vi "Homing.vi"(7 "Offset Home 2 RCM":dbl[](array[numeric])=[0.0, 0.0, 0.0, 0.0], 8 "error in":errorcluster, 9 "Stage PID Cluster":T2={"Stage Z PID"={"Kp"=0.0005, "Kd"=0.001, "Ki"=0.0}, "Stage Y PID"={"Kp"=0.0003, "Kd"=0.01, "Ki"=0.0}, "Stage X PID"={"Kp"=0.0003, "Kd"=0.01, "Ki"=0.0}}, 10 "L1 to L4 PID Cluster":T1={"L1 PID Gains"={"Kp"=0.005, "Kd"=0.5, "Ki"=0.0005}, "L2 PID Gains"={"Kp"=0.01, "Kd"=1.0, "Ki"=0.005}, "L3 PID Gains"={"Kp"=0.05, "Kd"=1.0, "Ki"=0.0005}, "L4 PID Gains"={"Kp"=0.1, "Kd"=0.1, "Ki"=0.0005}}, 11 "FPGA VI Reference In":refnum<k20>) -> (0 "error out":errorcluster, 1 "Last Stage Posit":dbl[](array[numeric]), 2 "Last L1 to L4 Posit":dbl[](array[numeric]), 3 "FPGA VI Reference Out":refnum<k20>)   [LabVIEW 2016]
uses:
  <vilib>/Platform/TimedLoop/XDataNode/timing_clust.ctl
  <vilib>/Platform/TimedLoop/XDataNode/nitl_modes.ctl
  <vilib>/Platform/TimedLoop/XDataNode/wakeup.ctl
  Library/KevinLibraryAll/labview2010/kevLib2010/Simple Filters/kDelay.vi
  Global Variables.vi
  <vilib>/Utility/error.llb/Error Cluster From Error Code.vi
  <vilib>/rvi/errors/niLvFpgaAdjustHostInterfaceError.vi
  <vilib>/platform/TimedLoop/XDataNode/XDataNode.xnode
  <vilib>/rvi/interface/nirviReadWriteControl/nirviReadWriteControl.xnode
  FPGA Bitfiles/IRISSTrack_FPGATarget2_IRISSFPGAIORIO_4NTO9ubhv-c.lvbitx
  IRISS_FPGA_IO_RIO.vi
  <vilib>/Platform/TimedLoop/XDataNode/XDNodeRunTimeDep.lvlib
  Library/KevinLibraryAll/labview2010/kevLib2010.lvlib
  Library/KevinLibraryAll/labview2011/kevLib2011.lvlib
  Library/KevinLibraryAll/labview/KevLib01.lvlib
  Library/jmslib.lvlib
  NiFpgaLv.dll
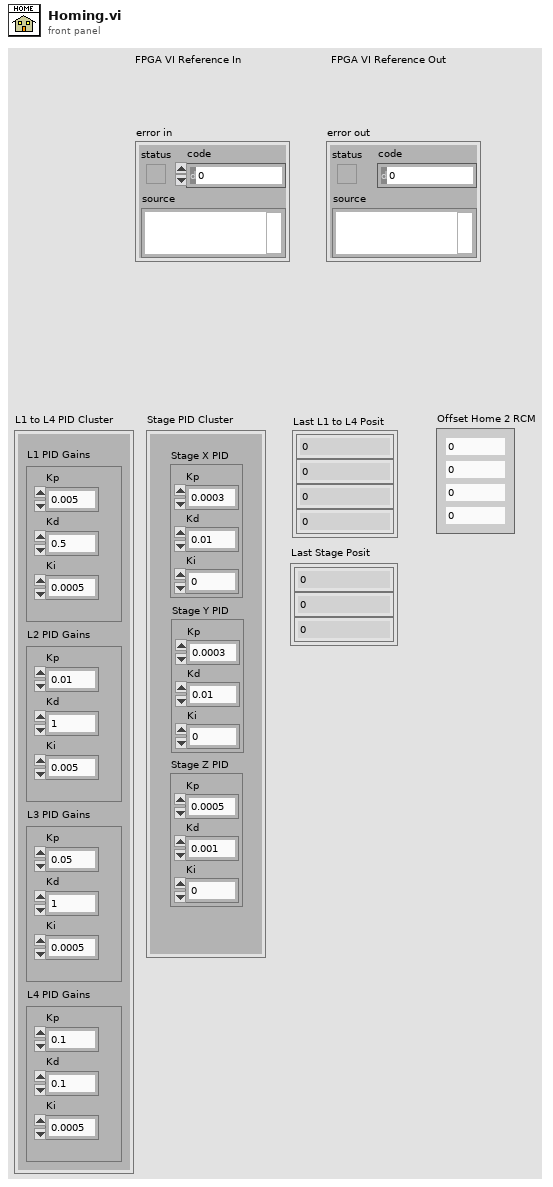
[diagram p1: front panel]
types:
  T1 = cluster{"L1 PID Gains":cluster{"Kp":dbl, "Kd":dbl, "Ki":dbl}, "L2 PID Gains":cluster{"Kp":dbl, "Kd":dbl, "Ki":dbl}, "L3 PID Gains":cluster{"Kp":dbl, "Kd":dbl, "Ki":dbl}, "L4 PID Gains":cluster{"Kp":dbl, "Kd":dbl, "Ki":dbl}}
  T2 = cluster{"Stage Z PID":cluster{"Kp":dbl, "Kd":dbl, "Ki":dbl}, "Stage Y PID":cluster{"Kp":dbl, "Kd":dbl, "Ki":dbl}, "Stage X PID":cluster{"Kp":dbl, "Kd":dbl, "Ki":dbl}}
  T3 = typedef "XDNodeRunTimeDep.lvlib/timing_clust.ctl" = cluster{"Expected End [f-1]":u64, "Actual End [f-1]":u64, "Finished Late? [f-1]":bool, "Expected End [i-1]":u64, "Actual End [i-1]":u64, "Finished Late? [i-1]":bool, "Expected Start [i]":u64, "Actual Start [i]":u64, "Expected Start [f]":u64, "Actual Start [f]":u64, "Source Name":string, "Structure Name":string, "Period":i64, "Deadline":i64, "Offset":i64, "Start":i64, "Priority":i32, "Timeout":i32, "Mode":T4, "Wakeup Reason":T5, "Error":errorcluster, "Source Type":string, "Secondary Source Type":string, "Global End Time":u64, "Global Start Time":u64, "Frame Duration":u64, "Iteration Duration":u64, "Assigned CPU":i32, "I/O Scan Engine Mode":u32}
  T4 = typedef "XDNodeRunTimeDep.lvlib/nitl_modes.ctl" = enum32{"No Change", "Process missed periods, maintain original phase", "Discard missed periods, maintain original phase", "Process missed periods, ignore original phase", "Discard missed periods, ignore original phase"}
  T5 = typedef "XDNodeRunTimeDep.lvlib/wakeup.ctl" = enum32{"Normal", "Aborted", "Asynchronous wakeup", "Timing source error", "Timed loop error", "Timeout"}
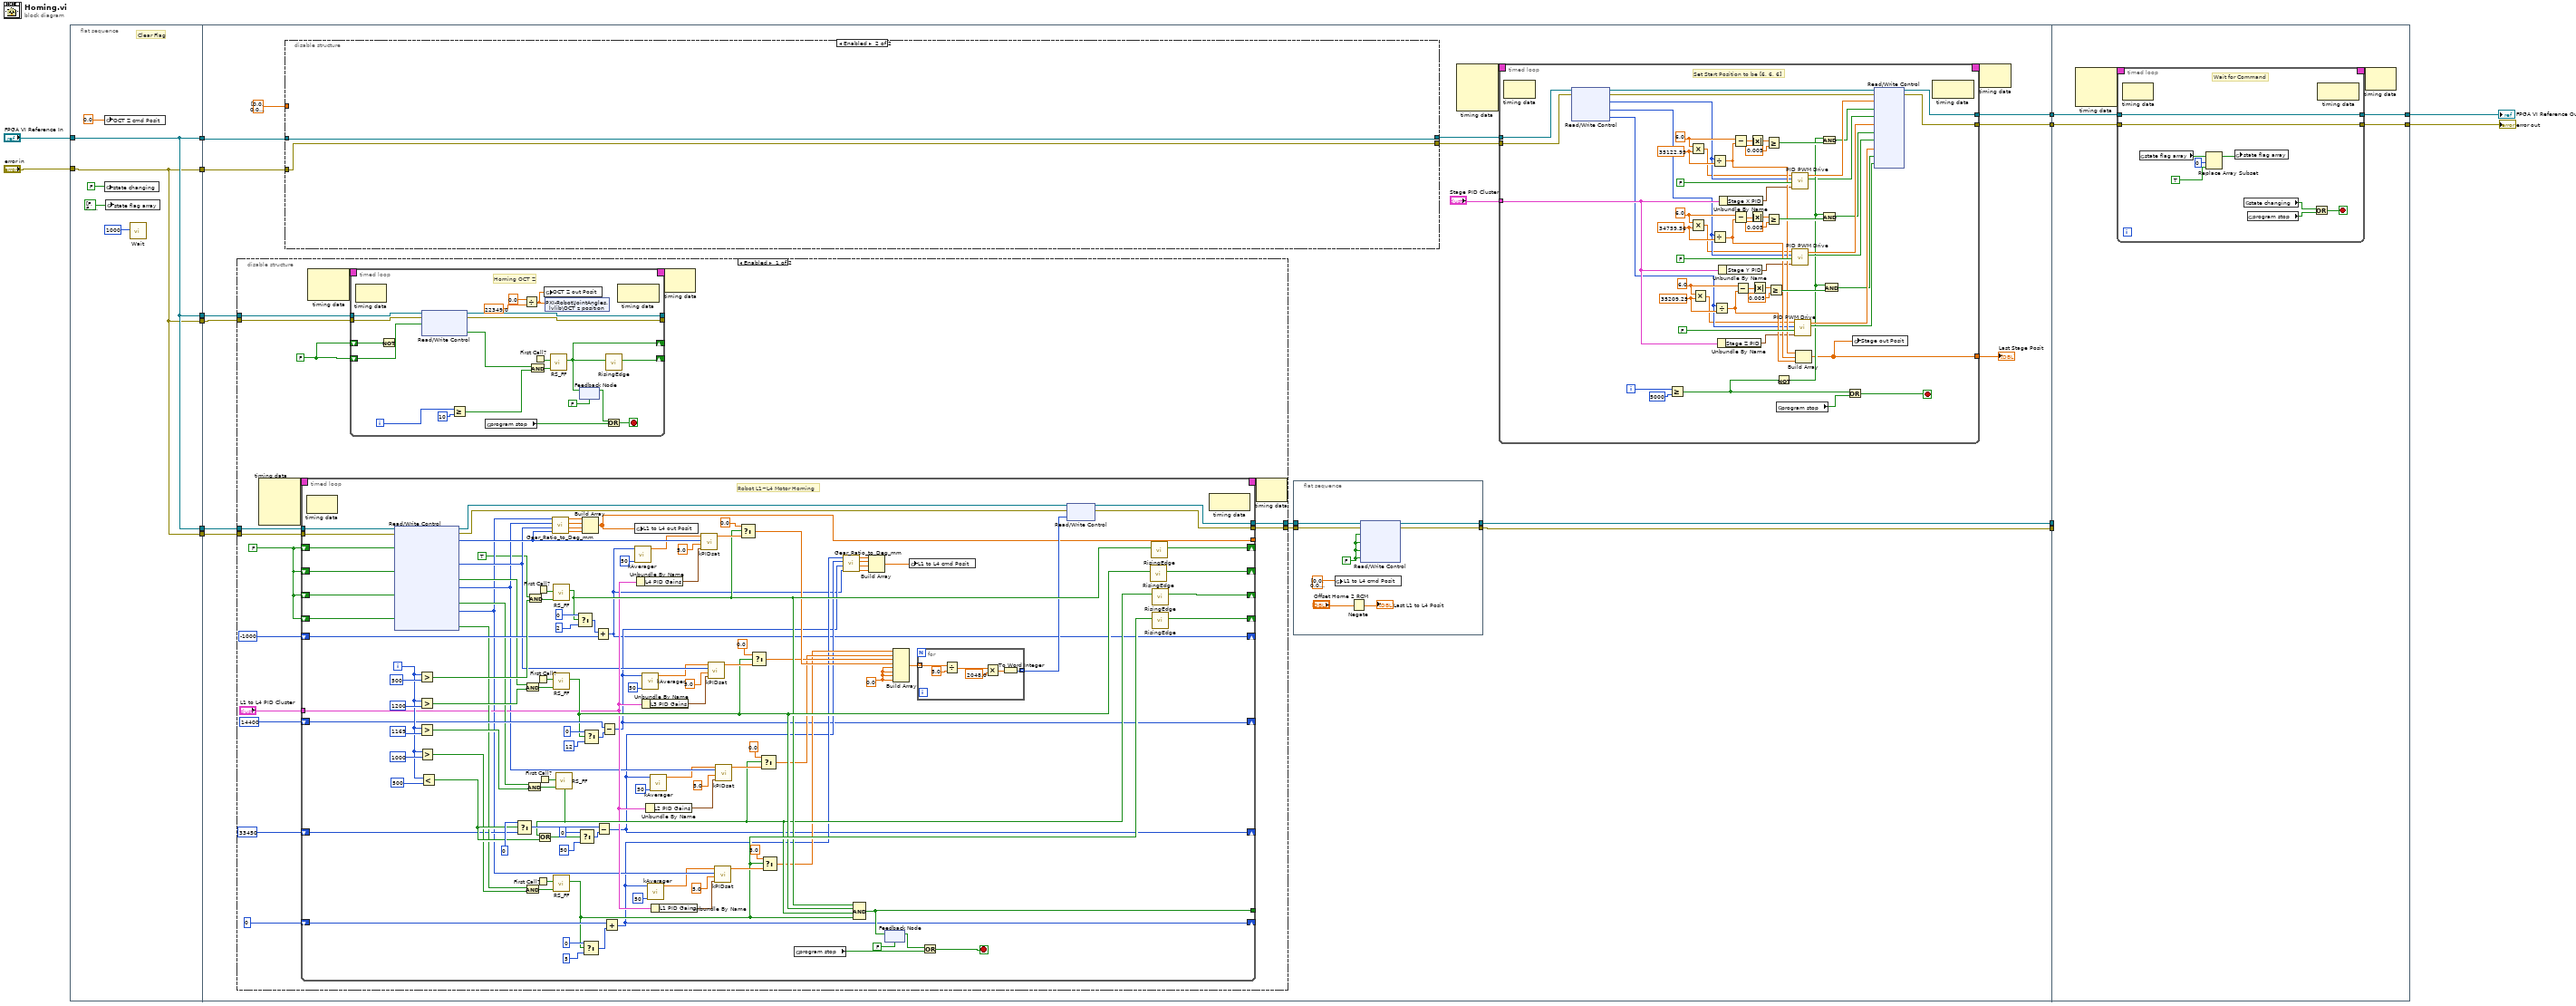
[diagram p0: block diagram]
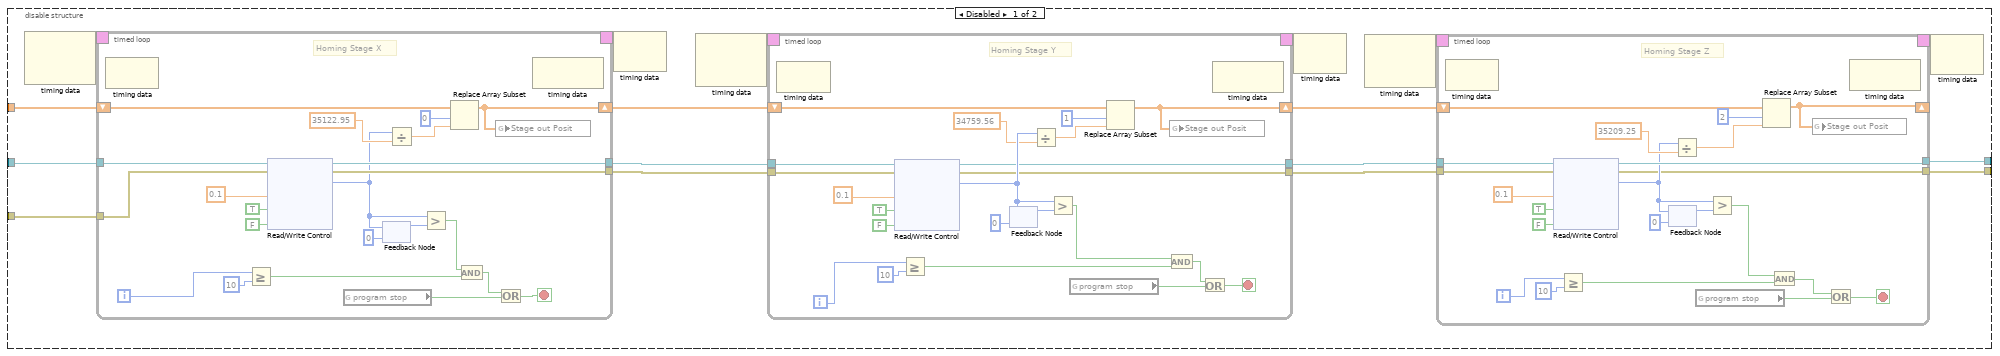
[diagram p3: hidden frame]
diagram:
  n1 = flat-sequence {
    tunnel: "FPGA VI Reference In" -> [w17]
    tunnel: "error in" -> [w16]
    tunnel: [w17] -> w14
    tunnel: [w17] -> w13
    tunnel: [w16] -> w12
    tunnel: [w16] -> w11
    tunnel: [w17] -> w6
    tunnel: [w16] -> w5
    tunnel: w14 -> [w37]
    tunnel: w13 -> [w36]
    tunnel: w12 -> [w35]
    tunnel: w11 -> [w34]
    tunnel: w6 -> [w33]
    tunnel: w5 -> [w32]
    tunnel: [w31] -> w4
    tunnel: [w30] -> w3
    tunnel: [w24] -> w2
    tunnel: [w23] -> w1
    tunnel: [w375] -> w8
    tunnel: [w374] -> w7
    tunnel: w4 -> [_]
    tunnel: w3 -> [_]
    tunnel: w2 -> [w373]
    tunnel: w1 -> [w372]
    frame #0 {
      # "Clear Flag"
      n2 = global write "Global Variables.vi" "OCT Z cmd Posit"(0.0) -> ()
      n3 = global write "Global Variables.vi" "state changing"(FALSE ("state changing")) -> ()
      n4 = global write "Global Variables.vi" "state flag array"(bool[] [FALSE, FALSE, FALSE, FALSE, FALSE, FALSE, FALSE, FALSE, FALSE] ("state flag array")) -> ()
      n5 = call "Wait"("Count(mSec)"=u32 1000 ("milliseconds to wait")) -> ()  [unwired: 1 out]
    }
    frame #1 {
      n6 = disable-structure shown="Enabled" {
        disable-tunnel: w36 -> [w52 _]
        disable-tunnel: w34 -> [w51 _]
        disable-tunnel: w33 -> [w50 _]
        disable-tunnel: w32 -> [w49 _]
        disable-tunnel: [w47 _] -> w22
        disable-tunnel: [w46 _] -> w21
        frame Enabled {
          w45 = FALSE ("Rising Edge")
          w48 = FALSE ("Rising Edge")
          n7 = node-c288() -> (w54:T3)  [unwired: 4 in]
          n8 = timed-loop {
            timing: w54 -> [_]
            timing-out: [_] -> w53
            tunnel: w52 -> [w171]
            tunnel: w51 -> [w170]
            shift-right: [w105] -> _
            shift-left: w45 -> [w169]
            shift-right: [w104] -> _
            shift-left: w45 -> [w168]
            shift-right: [w103] -> _
            shift-left: w45 -> [w167]
            shift-right: [w102] -> _
            shift-left: w45 -> [w166]
            shift-right: [w60] -> _
            shift-left: -1000 -> [w149]
            shift-right: [w61] -> _
            shift-left: 14400 -> [w141]
            shift-right: [w62] -> _
            shift-left: 33450 -> [w112]
            shift-right: [w63] -> _
            shift-left: 0 -> [w111]
            tunnel: [w106] -> _
            tunnel: [w86] -> w47
            tunnel: [w85] -> w46
            tunnel: "L1 to L4 PID Cluster" -> [w81]
            tunnel: [w59] -> _
            i -> [w151]
            stop <- w107 stop-if-true
            w97 = 0.0 ("element")
            # "Robot L1~L4 Motor Homing"
            n9 = node-c288() -> ()  [unwired: 1 in, 1 out]
            n10 = xnode "Read/Write Control"("FPGA VI Reference In"=w171, "error in"=w170, "Reset C1-4"=w169, "Reset C1-1"=w168, "Reset 3"=w167, "Reset 1"=w166) -> ("FPGA VI Reference Out"=w94:refnum<k20>, "error out"=w93:errorcluster, "32 bit Position C1-4"=w79:i32, "32 bit Position C1-1"=w78:i32, "Home L3"=w132:bool, "32 bit Position 3"=w77:i32, "Home L2"=w130:bool, "32 bit Position 1"=w76:i32, "Home L1"=w117:bool)  [unwired: 1 out]
            n11 = Greater?(x=w151, y=500) -> (0:w150:bool)
            n12 = Greater?(x=w151, y=1200) -> (0:w133:bool)
            n13 = Greater?(x=w151, y=1169) -> (0:w131:bool)
            n14 = Greater?(x=w151, y=1000) -> (0:w116:bool)
            n15 = Less?(x=w151, y=500) -> (x < y?=w123:bool)
            n16 = Select(t=0, s=w123, f=w112) -> (s? t:f=w128:i32)
            n17 = And(x=w132, y=w133) -> (x .and. y?=w142:bool)
            n18 = And(x=w117, y=w116) -> (x .and. y?=w118:bool)
            n19 = And(x=w130, y=w131) -> (x .and. y?=w135:bool)
            n20 = And(x=TRUE, y=w150) -> (x .and. y?=w162:bool)
            n21 = First Call?() -> (First Call?: T/F=w143:bool)
            n22 = First Call?() -> (First Call?: T/F=w119:bool)
            n23 = First Call?() -> (First Call?: T/F=w161:bool)
            n24 = First Call?() -> (First Call?: T/F=w134:bool)
            n25 = call "Gear_Ratio_to_Deg_mm.vi"("j4"=w79, "j3"=w78, "j2"=w77, "j1"=w76) -> ("theta 4"=w72:dbl, "theta 3"=w73:dbl, "theta 2"=w74:dbl, "theta 1"=w75:dbl)
            n26 = call "RS_FF.vi"("Set"=w162, "Reset"=w161) -> ("Result"=w99:bool)  [unwired: 9 in]
            n27 = call "RS_FF.vi"("Set"=w142, "Reset"=w143) -> ("Result"=w100:bool)  [unwired: 9 in]
            n28 = call "RS_FF.vi"("Set"=w118, "Reset"=w119) -> ("Result"=w101:bool)  [unwired: 9 in]
            n29 = call "RS_FF.vi"("Set"=w135, "Reset"=w134) -> ("Result"=w98:bool)  [unwired: 9 in]
            n30 = Or(x=w98, y=w123) -> (x .or. y?=w127:bool)
            n31 = Select(t=0, s=w99, f=2) -> (s? t:f=w163:i32)
            n32 = Select(t=0, s=w127, f=50) -> (s? t:f=w124:i32)
            n33 = Build Array(w75, w74, w73, w72) -> (w59:dbl[])
            n34 = Select(t=0, s=w101, f=5) -> (s? t:f=w122:i32)
            n35 = Select(t=0, s=w100, f=12) -> (s? t:f=w144:i32)
            n36 = Add(x=w163, y=w149) -> (x+y=w60:i32)
            n37 = Subtract(x=w128, y=w124) -> (x-y=w62:i32)
            n38 = Subtract(x=w141, y=w144) -> (x-y=w61:i32)
            n39 = Add(x=w111, y=w122) -> (x+y=w63:i32)
            n40 = call "kAverager.vi"("num avg"=50, "input"=w60) -> ("output"=w64:dbl)  [unwired: 9 in]
            n41 = global write "Global Variables.vi" "L1 to L4 out Posit"(w59) -> ()
            n42 = Unbundle By Name(w81) -> ("L4 PID Gains"=w84:cluster{"Kp":dbl, "Kd":dbl, "Ki":dbl})
            n43 = Unbundle By Name(w81) -> ("L3 PID Gains"=w83:cluster{"Kp":dbl, "Kd":dbl, "Ki":dbl})
            n44 = call "kAverager.vi"("num avg"=50, "input"=w61) -> ("output"=w65:dbl)  [unwired: 9 in]
            n45 = Unbundle By Name(w81) -> ("L2 PID Gains"=w82:cluster{"Kp":dbl, "Kd":dbl, "Ki":dbl})
            n46 = call "kAverager.vi"("num avg"=50, "input"=w63) -> ("output"=w67:dbl)  [unwired: 9 in]
            n47 = call "kAverager.vi"("num avg"=50, "input"=w62) -> ("output"=w66:dbl)  [unwired: 9 in]
            n48 = Unbundle By Name(w81) -> ("L1 PID Gains"=w80:cluster{"Kp":dbl, "Kd":dbl, "Ki":dbl})
            n49 = call "kPIDsat.vi"("PID Gains"=w84, "Sat Limit"=5.0, "Position"=w79, "Reference"=w64) -> ("Control"=w158:dbl)  [unwired: 7 in]
            n50 = call "kPIDsat.vi"("PID Gains"=w83, "Sat Limit"=5.0, "Position"=w78, "Reference"=w65) -> ("Control"=w139:dbl)  [unwired: 7 in]
            n51 = call "kPIDsat.vi"("PID Gains"=w80, "Sat Limit"=5.0, "Position"=w76, "Reference"=w67) -> ("Control"=w113:dbl)  [unwired: 7 in]
            n52 = call "kPIDsat.vi"("PID Gains"=w82, "Sat Limit"=5.0, "Position"=w77, "Reference"=w66) -> ("Control"=w138:dbl)  [unwired: 7 in]
            n53 = Select(t=0.0, s=w99, f=w158) -> (s? t:f=w92:dbl)
            n54 = Select(t=0.0 ("element"), s=w100, f=w139) -> (s? t:f=w91:dbl)
            n55 = Select(t=0.0 ("element"), s=w98, f=w138) -> (s? t:f=w90:dbl)
            n56 = Select(t=3.0 ("element"), s=w101, f=w113) -> (s? t:f=w89:dbl)
            n57 = global read "Global Variables.vi" "program stop"() -> (w108:bool)
            n58 = call "Gear_Ratio_to_Deg_mm.vi"("j4"=w60, "j3"=w61, "j2"=w62, "j1"=w63) -> ("theta 4"=w68:dbl, "theta 3"=w69:dbl, "theta 2"=w70:dbl, "theta 1"=w71:dbl)
            n59 = Compound Arithmetic op=AND(w99, w100, w98, w101) -> (w106:bool)
            n60 = Build Array(w71, w70, w69, w68) -> (w58:dbl[])
            n61 = feedback #1(FALSE) -> (w109:bool)
            n62 = feedback-in #1(w106) -> ()
            n63 = Build Array(w89, w90, w91, w92, w97, w97, w97, w97) -> (w96:dbl[])
            n64 = global write "Global Variables.vi" "L1 to L4 cmd Posit"(w58) -> ()
            n65 = for {
              tunnel: [w175] -> w95 mode=indexing
              tunnel: w96 -> [w174] mode=indexing
              n66 = Divide(x=w174, y=5.0) -> (x/y=w177:dbl)
              n67 = Multiply(x=w177, y=2048.0) -> (x*y=w176:dbl)
              n68 = To Word Integer(number=w176) -> (16bit integer=w175:i16)
            }
            n69 = Or(x=w109, y=w108) -> (x .or. y?=w107:bool)
            n70 = xnode "Read/Write Control"("FPGA VI Reference In"=w94, "error in"=w93, "AO"=w95) -> ("FPGA VI Reference Out"=w86:refnum<k20>, "error out"=w85:errorcluster)
            n71 = call "RisingEdge.vi"("Signal In"=w100) -> ("Rising Edge"=w104:bool)  [unwired: 10 in]
            n72 = call "RisingEdge.vi"("Signal In"=w99) -> ("Rising Edge"=w105:bool)  [unwired: 10 in]
            n73 = call "RisingEdge.vi"("Signal In"=w98) -> ("Rising Edge"=w103:bool)  [unwired: 10 in]
            n74 = call "RisingEdge.vi"("Signal In"=w101) -> ("Rising Edge"=w102:bool)  [unwired: 10 in]
            n75 = node-c288() -> ()  [unwired: 1 in, 1 out]
          }
          n76 = node-c288() -> (w56:T3)  [unwired: 2 in]
          n77 = timed-loop {
            timing: w56 -> [_]
            timing-out: [_] -> w55
            tunnel: w50 -> [w199]
            tunnel: w49 -> [w198]
            tunnel: [w197] -> _
            tunnel: [w196] -> _
            shift-right: [w191] -> _
            shift-left: w48 -> [w193]
            shift-right: [w187] -> _
            shift-left: w48 -> [w185]
            i -> [w200]
            stop <- w194 stop-if-true
            # "Homing OCT Z"
            n78 = node-c288() -> ()  [unwired: 1 in, 1 out]
            n79 = Not(x=w185) -> ()  [unwired: 1 out]
            n80 = xnode "Read/Write Control"("FPGA VI Reference In"=w199, "error in"=w198, "Reset 14"=w193) -> ("FPGA VI Reference Out"=w197:refnum<k20>, "error out"=w196:errorcluster, "Home OCT z"=w192:bool)
            n81 = Greater Or Equal?(x=w200, y=10) -> (x >= y?=w202:bool)
            n82 = global read "Global Variables.vi" "program stop"() -> (w195:bool)
            n83 = Divide(x=0.0, y=22349.0) -> (x/y=w183:dbl)
            n84 = And(x=w192, y=w202) -> (x .and. y?=w189:bool)
            n85 = First Call?() -> (First Call?: T/F=w190:bool)
            n86 = global write "Global Variables.vi" "OCT Z out Posit"(w183) -> ()
            n87 = shared-variable "PXI-Robot\\JointAngles.lvlib\\OCT z position"(w183) -> ()  [unwired: 1 in, 1 out]
            n88 = call "RS_FF.vi"("Set"=w189, "Reset"=w190) -> ("Result"=w187:bool)  [unwired: 9 in]
            n89 = feedback #2(FALSE) -> (w186:bool)
            n90 = feedback-in #2(w187) -> ()
            n91 = call "RisingEdge.vi"("Signal In"=w187) -> ("Rising Edge"=w191:bool)  [unwired: 10 in]
            n92 = Or(x=w186, y=w195) -> (x .or. y?=w194:bool)
            n93 = node-c288() -> ()  [unwired: 1 in, 1 out]
          }
          n94 = node-c288(w55) -> ()  [unwired: 1 out]
          n95 = node-c288(w53) -> ()  [unwired: 1 out]
        }
        frame Disabled {
        }
      }
      n96 = disable-structure shown="Enabled" {
        disable-tunnel: [w217 w303] -> w39
        disable-tunnel: [w216 w302] -> w38
        disable-tunnel: w37 -> [w215 w303]
        disable-tunnel: w35 -> [w214 w302]
        disable-tunnel: dbl[] [0.0, 0.0, 0.0] ("Stage Posit Array") -> [w207 _]
        frame Disabled {
          n97 = node-c288() -> (w219:T3)  [unwired: 2 in]
          n98 = timed-loop {
            timing: w219 -> [_]
            timing-out: [_] -> w218
            tunnel: w215 -> [w235]
            tunnel: w214 -> [w234]
            tunnel: [w233] -> w210
            tunnel: [w232] -> w209
            shift-right: [w224] -> w208
            shift-left: w207 -> [w226]
            i -> [w236]
            stop <- w229 stop-if-true
            # "Homing Stage X"
            n99 = node-c288() -> ()  [unwired: 1 in, 1 out]
            n100 = Greater Or Equal?(x=w236, y=10) -> (x >= y?=w245:bool)
            n101 = xnode "Read/Write Control"("FPGA VI Reference In"=w235, "error in"=w234, "X DC"=0.1 ("y"), "INHB X"=TRUE ("INHB Y"), "DIR X"=FALSE ("INHB Y")) -> ("FPGA VI Reference Out"=w233:refnum<k20>, "error out"=w232:errorcluster, "Position X"=w225:i32)
            n102 = global read "Global Variables.vi" "program stop"() -> (w231:bool)
            n103 = feedback #3(0 ("Position Y")) -> (w242:i32)
            n104 = feedback-in #3(w225) -> ()
            n105 = Divide(x=w225, y=35122.95) -> (x/y=w227:dbl)
            n106 = Greater?(x=w225, y=w242) -> (0:w243:bool)
            n107 = Replace Array Subset(array=w226, new element=w227, index=0) -> (w224:dbl[])
            n108 = And(x=w243, y=w245) -> (x .and. y?=w230:bool)
            n109 = global write "Global Variables.vi" "Stage out Posit"(w224) -> ()
            n110 = Or(x=w230, y=w231) -> (x .or. y?=w229:bool)
            n111 = node-c288() -> ()  [unwired: 1 in, 1 out]
          }
          n112 = node-c288(w218) -> ()  [unwired: 1 out]
          n113 = node-c288() -> (w221:T3)  [unwired: 2 in]
          n114 = timed-loop {
            timing: w221 -> [_]
            timing-out: [_] -> w220
            tunnel: w210 -> [w260]
            tunnel: w209 -> [w261]
            tunnel: [w258] -> w213
            tunnel: [w257] -> w212
            shift-right: [w250] -> w211
            shift-left: w208 -> [w251]
            i -> [w259]
            stop <- w256 stop-if-true
            # "Homing Stage Y"
            n115 = node-c288() -> ()  [unwired: 1 in, 1 out]
            n116 = xnode "Read/Write Control"("FPGA VI Reference In"=w260, "error in"=w261, "Y DC"=0.1 ("y"), "INHB Y"=TRUE, "DIR Y"=FALSE ("INHB Y")) -> ("FPGA VI Reference Out"=w258:refnum<k20>, "error out"=w257:errorcluster, "Position Y"=w268:i32)
            n117 = Greater Or Equal?(x=w259, y=10) -> (x >= y?=w271:bool)
            n118 = feedback #4(0 ("Position Y")) -> (w267:i32)
            n119 = feedback-in #4(w268) -> ()
            n120 = Divide(x=w268, y=34759.56) -> (x/y=w252:dbl)
            n121 = Greater?(x=w268, y=w267) -> (0:w269:bool)
            n122 = global read "Global Variables.vi" "program stop"() -> (w254:bool)
            n123 = Replace Array Subset(array=w251, new element=w252, index=1) -> (w250:dbl[])
            n124 = And(x=w269, y=w271) -> (x .and. y?=w255:bool)
            n125 = global write "Global Variables.vi" "Stage out Posit"(w250) -> ()
            n126 = Or(x=w255, y=w254) -> (x .or. y?=w256:bool)
            n127 = node-c288() -> ()  [unwired: 1 in, 1 out]
          }
          n128 = node-c288(w220) -> ()  [unwired: 1 out]
          n129 = node-c288() -> (w223:T3)  [unwired: 2 in]
          n130 = timed-loop {
            timing: w223 -> [_]
            timing-out: [_] -> w222
            tunnel: w213 -> [w297]
            tunnel: [w296] -> w217
            tunnel: w212 -> [w284]
            tunnel: [w283] -> w216
            shift-right: [w276] -> _
            shift-left: w211 -> [w277]
            i -> [w287]
            stop <- w281 stop-if-true
            # "Homing Stage Z"
            n131 = node-c288() -> ()  [unwired: 1 in, 1 out]
            n132 = xnode "Read/Write Control"("FPGA VI Reference In"=w297, "error in"=w284, "Z DC"=0.1 ("y"), "INHB Z"=TRUE ("INHB Y"), "DIR Z"=FALSE ("INHB Y")) -> ("FPGA VI Reference Out"=w296:refnum<k20>, "error out"=w283:errorcluster, "Position Z"=w289:i32)
            n133 = Greater Or Equal?(x=w287, y=10) -> (x >= y?=w285:bool)
            n134 = feedback-in #5(w289) -> ()
            n135 = feedback #5(0 ("Position Y")) -> (w290:i32)
            n136 = Divide(x=w289, y=35209.25) -> (x/y=w278:dbl)
            n137 = global read "Global Variables.vi" "program stop"() -> (w282:bool)
            n138 = Greater?(x=w289, y=w290) -> (0:w288:bool)
            n139 = Replace Array Subset(array=w277, new element=w278, index=2) -> (w276:dbl[])
            n140 = And(x=w288, y=w285) -> (x .and. y?=w280:bool)
            n141 = global write "Global Variables.vi" "Stage out Posit"(w276) -> ()
            n142 = Or(x=w280, y=w282) -> (x .or. y?=w281:bool)
            n143 = node-c288() -> ()  [unwired: 1 in, 1 out]
          }
          n144 = node-c288(w222) -> ()  [unwired: 1 out]
        }
        frame Enabled {
        }
      }
      n145 = flat-sequence {
        tunnel: w22 -> [w310]
        tunnel: w21 -> [w309]
        tunnel: [w305] -> w31
        tunnel: [w304] -> w30
        frame #0 {
          w311 = FALSE ("Reset 1")
          n146 = global write "Global Variables.vi" "L1 to L4 cmd Posit"(dbl[] [0.0, 0.0, 0.0, 0.0] ("L1 to L4 cmd Posit")) -> ()
          n147 = Negate(x="Offset Home 2 RCM") -> (-x=→"Last L1 to L4 Posit":dbl[])
          n148 = xnode "Read/Write Control"("FPGA VI Reference In"=w310, "error in"=w309, "Reset C1-4"=w311, "Reset C1-1"=w311, "Reset 3"=w311, "Reset 1"=w311) -> ("FPGA VI Reference Out"=w305:refnum<k20>, "error out"=w304:errorcluster)
        }
      }
      n149 = node-c288() -> (w29:T3)  [unwired: 4 in]
      n150 = timed-loop {
        timing: w29 -> [_]
        timing-out: [_] -> w28
        tunnel: w39 -> [w332]
        tunnel: w38 -> [w333]
        tunnel: "Stage PID Cluster" -> [w341]
        tunnel: [w314] -> w26
        tunnel: [w313] -> w24
        tunnel: [w312] -> w23
        i -> [w367]
        stop <- w331 stop-if-true
        w344 = 6.0 ("y")
        w347 = 35209.25 ("y")
        w358 = 6.0 ("y")
        w355 = 34759.56 ("y")
        w359 = 6.0 ("y")
        w362 = 35122.95 ("y")
        # "Set Start Position to be [6, 6, 6]"
        n151 = node-c288() -> ()  [unwired: 1 in, 1 out]
        n152 = xnode "Read/Write Control"("FPGA VI Reference In"=w332, "error in"=w333) -> ("FPGA VI Reference Out"=w335:refnum<k20>, "error out"=w334:errorcluster, "Position X"=w330:i32, "Position Y"=w329:i32, "Position Z"=w328:i32)
        n153 = Greater Or Equal?(x=w367, y=5000) -> (x >= y?=w320:bool)
        n154 = Multiply(x=w359, y=w362) -> (x*y=w327:dbl)
        n155 = Multiply(x=w358, y=w355) -> (x*y=w326:dbl)
        n156 = Multiply(x=w344, y=w347) -> (x*y=w325:dbl)
        n157 = Divide(x=w330, y=w362) -> (x/y=w340:dbl)
        n158 = Divide(x=w329, y=w355) -> (x/y=w339:dbl)
        n159 = Divide(x=w328, y=w347) -> (x/y=w338:dbl)
        n160 = Unbundle By Name(w341) -> ("Stage Z PID"=w336:cluster{"Kp":dbl, "Kd":dbl, "Ki":dbl})
        n161 = Unbundle By Name(w341) -> ("Stage Y PID"=w337:cluster{"Kp":dbl, "Kd":dbl, "Ki":dbl})
        n162 = Unbundle By Name(w341) -> ("Stage X PID"=w321:cluster{"Kp":dbl, "Kd":dbl, "Ki":dbl})
        n163 = Subtract(x=w359, y=w340) -> (x-y=w363:dbl)
        n164 = Subtract(x=w358, y=w339) -> (x-y=w354:dbl)
        n165 = Subtract(x=w344, y=w338) -> (x-y=w348:dbl)
        n166 = Absolute Value(x=w363) -> (abs(x)=w364:dbl)
        n167 = Absolute Value(x=w354) -> (abs(x)=w353:dbl)
        n168 = Absolute Value(x=w348) -> (abs(x)=w349:dbl)
        n169 = Greater Or Equal?(x=w364, y=0.005) -> (x >= y?=w360:bool)
        n170 = Greater Or Equal?(x=w353, y=0.005) -> (x >= y?=w357:bool)
        n171 = Greater Or Equal?(x=w349, y=0.005) -> (x >= y?=w345:bool)
        n172 = Not(x=w320) -> (.not. x?=w319:bool)
        n173 = global read "Global Variables.vi" "program stop"() -> (w342:bool)
        n174 = call "PID PWM Drive.vi"("PID Gains"=w321, "Reverse Motor?"=FALSE, "Encoder Position"=w330, "Reference"=w327) -> ("Direction"=w317:bool, "Duty Cycle"=w324:dbl)  [unwired: 5 in, 1 out]
        n175 = call "PID PWM Drive.vi"("PID Gains"=w337, "Reverse Motor?"=FALSE, "Encoder Position"=w329, "Reference"=w326) -> ("Direction"=w351:bool, "Duty Cycle"=w323:dbl)  [unwired: 5 in, 1 out]
        n176 = call "PID PWM Drive.vi"("PID Gains"=w336, "Reverse Motor?"=FALSE, "Encoder Position"=w328, "Reference"=w325) -> ("Direction"=w343:bool, "Duty Cycle"=w322:dbl)  [unwired: 5 in, 1 out]
        n177 = Build Array(w340, w339, w338) -> (w314:dbl[])
        n178 = And(x=w319, y=w360) -> (x .and. y?=w318:bool)
        n179 = And(x=w319, y=w357) -> (x .and. y?=w316:bool)
        n180 = And(x=w319, y=w345) -> (x .and. y?=w315:bool)
        n181 = Or(x=w320, y=w342) -> (x .or. y?=w331:bool)
        n182 = global write "Global Variables.vi" "Stage out Posit"(w314) -> ()
        n183 = xnode "Read/Write Control"("FPGA VI Reference In"=w335, "error in"=w334, "X DC"=w324, "INHB X"=w318, "DIR X"=w317, "Y DC"=w323, "INHB Y"=w316, "DIR Y"=w351, "Z DC"=w322, "INHB Z"=w315, "DIR Z"=w343) -> ("FPGA VI Reference Out"=w313:refnum<k20>, "error out"=w312:errorcluster)
        n184 = node-c288() -> ()  [unwired: 1 in, 1 out]
      }
      "Last Stage Posit" <- w26
      n185 = node-c288(w28) -> ()  [unwired: 1 out]
    }
    frame #2 {
      n186 = node-c288() -> (w377:T3)  [unwired: 3 in]
      n187 = timed-loop {
        timing: w377 -> [_]
        timing-out: [_] -> w376
        tunnel: w373 -> [w380]
        tunnel: [w380] -> w375
        tunnel: [w379] -> w374
        tunnel: w372 -> [w379]
        stop <- w378 stop-if-true
        # "Wait for Command"
        n188 = node-c288() -> ()  [unwired: 1 in, 1 out]
        n189 = global read "Global Variables.vi" "state flag array"() -> (w384:bool[])
        n190 = Replace Array Subset(array=w384, new element=TRUE ("new element/subarray"), index=0) -> (w383:bool[])
        n191 = global write "Global Variables.vi" "state flag array"(w383) -> ()
        n192 = global read "Global Variables.vi" "state changing"() -> (w386:bool)
        n193 = global read "Global Variables.vi" "program stop"() -> (w385:bool)
        n194 = Or(x=w386, y=w385) -> (x .or. y?=w378:bool)
        n195 = node-c288() -> ()  [unwired: 1 in, 1 out]
      }
      n196 = node-c288(w376) -> ()  [unwired: 1 out]
    }
  }
  "FPGA VI Reference Out" <- w8
  "error out" <- w7
